vi "Save Framework Configuration.vi"(7 "overwrite? (T)":bool=TRUE, 8 "error in (no error)":errorcluster, 9 "framework configuration":T1, 10 "path in":path, 11 "Configuration in":refnum<class "Configuration.lvclass">) -> (0 "error out":errorcluster, 3 "Configuration out":refnum<class "Configuration.lvclass">)   [LabVIEW 2017, in "DSF Core.lvlib" / "Configuration Session.lvclass"]
uses:
  Configuration Session.lvclass
  JSON Builder/JSON Builder.lvclass
  Configuration.lvclass
  Typedefs/DSF Timing Info.ctl
  DSF Core.lvlib
  Typedefs/DSF Settings Info.ctl
  Typedefs/DSF Engine Plugin Thread Configuration.ctl
  Typedefs/DSF Direction.ctl
  Typedefs/DSF Byte Order.ctl
  Typedefs/DSF Data Type.ctl
  Typedefs/DSF Engine Channel Configuration.ctl
  Typedefs/DSF Engine Transfer Configuration.ctl
  Typedefs/DSF Timeout Behavior.ctl
  Typedefs/DSF Engine Transfer Group Configuration.ctl
  Typedefs/DSF Engine Plugin Configuration.ctl
  Typedefs/DSF Engine Framework Configuration.ctl
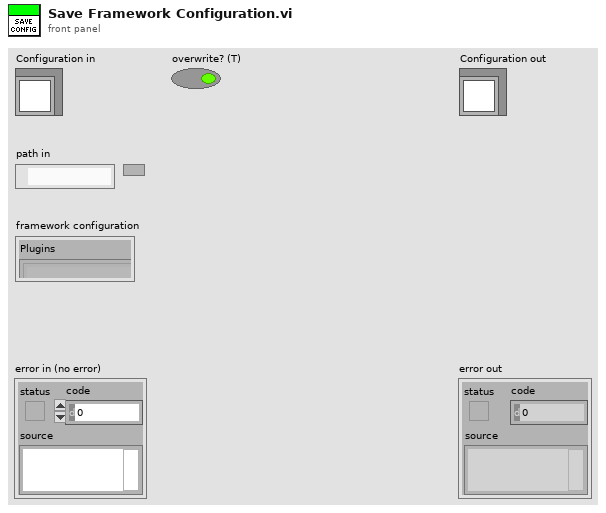
[diagram p1: front panel]
types:
  T1 = typedef "DSF Core.lvlib/DSF Engine Framework Configuration.ctl" = cluster{"Plugins":T2[]}
  T2 = typedef "DSF Core.lvlib/DSF Engine Plugin Configuration.ctl" = cluster{"name":string, "components":string[], "cycle timing":T3, "threads":T4[], "Transfer Groups":T6[], "settings":T5}
  T3 = typedef "DSF Core.lvlib/DSF Timing Info.ctl" = cluster{"priority":u64, "decimation":u64, "offset":u64}
  T4 = typedef "DSF Core.lvlib/DSF Engine Plugin Thread Configuration.ctl" = cluster{"buffer converter settings":T5, "transceiver settings":T5, "custom settings":T5, "processor":i32, "priority offset":i16}
  T5 = typedef "DSF Core.lvlib/DSF Settings Info.ctl" = cluster{"key":string, "value":string}[]
  T6 = typedef "DSF Core.lvlib/DSF Engine Transfer Group Configuration.ctl" = cluster{"name":string, "direction":T7, "cycle timing":T3, "thread index":i32, "settings":T5, "Transfers":T8[], "timeout behavior":T12}
  T7 = typedef "DSF Core.lvlib/DSF Direction.ctl" = enum8{"Tx", "Rx"}
  T8 = typedef "DSF Core.lvlib/DSF Engine Transfer Configuration.ctl" = cluster{"name":string, "byte order":T9, "settings":T5, "channels":T10[]}
  T9 = typedef "DSF Core.lvlib/DSF Byte Order.ctl" = enum8{"big-endian", "little-endian"}
  T10 = typedef "DSF Core.lvlib/DSF Engine Channel Configuration.ctl" = cluster{"string offset":u64, "string data type":T11, "engine data type":T11, "name":string, "settings":T5, "units":string}
  T11 = typedef "DSF Core.lvlib/DSF Data Type.ctl" = enum8{"Bool", "SGL", "DBL", "I8", "I16", "I32", "I64", "U8", "U16", "U32", "U64"}
  T12 = typedef "DSF Core.lvlib/DSF Timeout Behavior.ctl" = enum8{"Increment Late Count", "Throw Error"}
  T13 = enum16{"open", "replace", "create", "open or create", "replace or create", "replace or create with confirmation"}
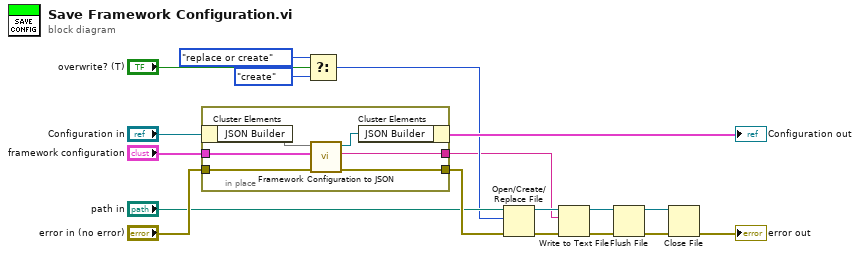
[diagram p0: block diagram]
diagram:
  n1 = in-place {
    in-place-border: [w24] -> w9
    in-place-border: "error in (no error)" -> [w21]
    in-place-border: [w20] -> w1
    in-place-border: "framework configuration" -> [w19]
    n2 = in-place-cluster #1("Configuration in") -> ("JSON Builder"=w23)
    n3 = call-dynamic "Framework Configuration to JSON.vi"("error in (no error)"=w21, "framework configuration"=w19, "JSON Builder in"=w23) -> ("error out"=w24:errorcluster, "JSON string"=w20:string, "JSON Builder out"=w22:refnum<class "JSON Builder.lvclass">)  [unwired: 6 in]
    n4 = in-place-cluster #1("JSON Builder"=w22) -> (→"Configuration out":cluster{})
  }
  n5 = Select(t=T13."replace or create" ("operation (0:open)"), s="overwrite? (T)", f=T13."create") -> (s? t:f=w5:T13)
  n6 = Open/Create/Replace File(file path (use dialog)="path in", error in=w9, operation (0:open)=w5) -> (refnum out=w18:refnum<file>, error out=w17:errorcluster)  [unwired: 3 in, 1 out]
  n7 = Write to Text File(file (use dialog)=w18, text=w1, error in=w17) -> (refnum out=w3:refnum<file>, error out=w16:errorcluster)  [unwired: 1 in, 1 out]
  n8 = Flush File(refnum=w3, error in=w16) -> (refnum out=w2:refnum<file>, error out=w4:errorcluster)
  n9 = Close File(refnum=w2, error in=w4) -> (error out=→"error out":errorcluster)  [unwired: 1 out]
